vi "myRIO__TCP_readAccumParse_removeInvalidChar.vi"(11 "input_string":string) -> (1 "output_droppedChar":bool, 2 "output_stringSize":i32, 3 "output_string":string)   [LabVIEW 2014]
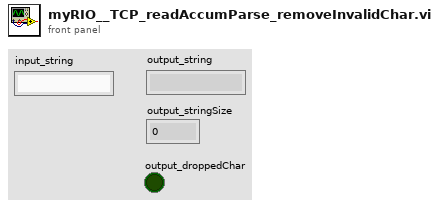
[diagram p1: front panel]
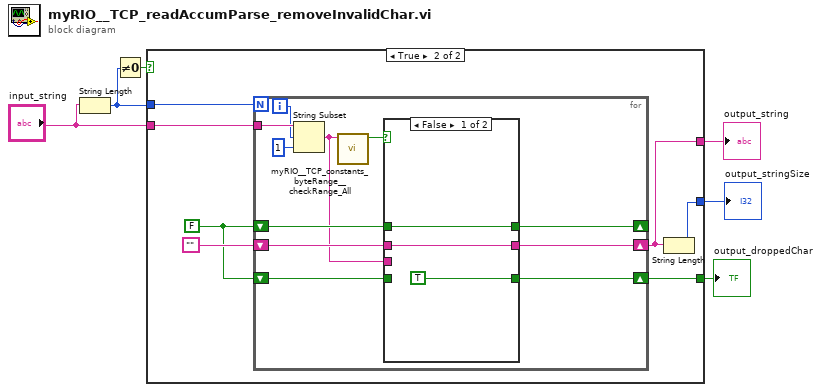
[diagram p0: block diagram]
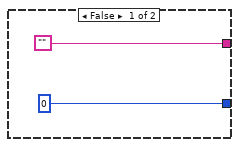
[diagram p2: hidden frame]
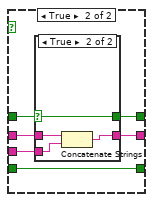
[diagram p3: hidden frame]
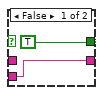
[diagram p4: hidden frame]
diagram:
  n1 = String Length(string="input_string") -> (length=w6:i32)
  n2 = Not Equal To 0?(x=w6) -> (x != 0?=w5:bool)
  n3 = case shown="True" w5 {
    tunnel: w6 -> [_ w15]
    tunnel: "input_string" -> [_ w14]
    tunnel: ["" w11] -> w3
    tunnel: [0 w12] -> w2
    tunnel: [_ w9] -> w1
    frame False {
    }
    frame True {
      w10 = FALSE
      n4 = for {
        N: w15 -> [_]
        tunnel: w14 -> [w26]
        shift-right: [w20] -> _
        shift-left: w10 -> [w21]
        shift-right: [w18] -> w11
        shift-left: "" -> [w22]
        shift-right: [w16] -> w9
        shift-left: w10 -> [w17]
        i -> [w25]
        n5 = String Subset(string=w26, offset (0)=w25, length (rest)=1 ("length (rest)")) -> (substring=w19:string)
        n6 = call "myRIO__TCP_constants_byteRange__checkRange_All.vi"("input_char"=w19) -> ("output_inRange"=w23:bool)  [unwired: 10 in]
        n7 = case shown="False" w23 {
          tunnel: w22 -> [w28 w32]
          tunnel: w21 -> [w29 w35]
          tunnel: [w29 w34] -> w20
          tunnel: w19 -> [_ w33]
          tunnel: [w28 w31] -> w18
          tunnel: w17 -> [_ w30]
          tunnel: [TRUE w30] -> w16
          frame False {
          }
          frame True {
            n8 = case shown="True" w35 {
              selector: w35 -> [_ w41]
              tunnel: [TRUE w41] -> w34
              tunnel: w33 -> [w36 w40]
              tunnel: w32 -> [_ w39]
              tunnel: [w36 w38] -> w31
              frame False {
              }
              frame True {
                n9 = Concatenate Strings(w39, w40) -> (w38:string)
              }
            }
          }
        }
      }
      n10 = String Length(string=w11) -> (length=w12:i32)
    }
  }
  "output_string" <- w3
  "output_stringSize" <- w2
  "output_droppedChar" <- w1
